vi "Menu_ItemName.vi"(7 "Ctrl":string, 8 "error in (no error)":errorcluster, 10 "DB Ref":T1, 11 "String":string) -> (0 "error out":errorcluster)   [LabVIEW 2017, in "tagdb-UIStateExpr Operations.lvlib"]
uses:
  tagdb-UIStateExpr Operations.lvlib
  <userlib>/_NEVSTOP/TagDB/Typedef/TagDB.ctl
  00d0da00-135c-4b50-b029-f1f1f0d03544.vi
  4c542a80-f847-4821-836c-1c9f0a826a9d.vi
  00d0da00-135c-4b50-b029-f1f1f0d03544.vi/1b47866c-8e2d-43a7-815f-8cf18635e5a1.vi
  4c542a80-f847-4821-836c-1c9f0a826a9d.vi/1b47866c-8e2d-43a7-815f-8cf18635e5a1.vi
  <userlib>/_NEVSTOP/TagDB/_Support/Change Detector/TagDB dbChanged.vi
  <userlib>/_NEVSTOP/TagDB/_Support/Error/_Clear Errors.vi
  00d0da00-135c-4b50-b029-f1f1f0d03544.vi/1b47866c-8e2d-43a7-815f-8cf18635e5a1.vi/29b2ea6d-6d7f-4e4a-ad31-a5cb760462c7.vi
  <userlib>/_NEVSTOP/TagDB/API/TagDB-Status.vi
  4c542a80-f847-4821-836c-1c9f0a826a9d.vi/1b47866c-8e2d-43a7-815f-8cf18635e5a1.vi/29b2ea6d-6d7f-4e4a-ad31-a5cb760462c7.vi
  <userlib>/_NEVSTOP/TagDB/_Support/Change Detector/TagDB ChangeFlag.vi
  <userlib>/_NEVSTOP/TagDB/_Support/DataAccess/_NameCacher.vi
  <userlib>/_NEVSTOP/TagDB/_Support/Error/_[error50002]Invalid DataType.vi
  <userlib>/_NEVSTOP/TagDB/_Support/Error/_[error50000]Invalid DB REF.vi
  <userlib>/_NEVSTOP/TagDB/_Support/DataAccess/TagDB Ref to DVR.vi
  <userlib>/_NEVSTOP/TagDB/_Support/URL/TRIM-BOTH-SPACE.vi
  <userlib>/_NEVSTOP/TagDB/_Support/Error/_Build Error Cluster.vi
  <userlib>/_NEVSTOP/TagDB/TagDB.lvlib
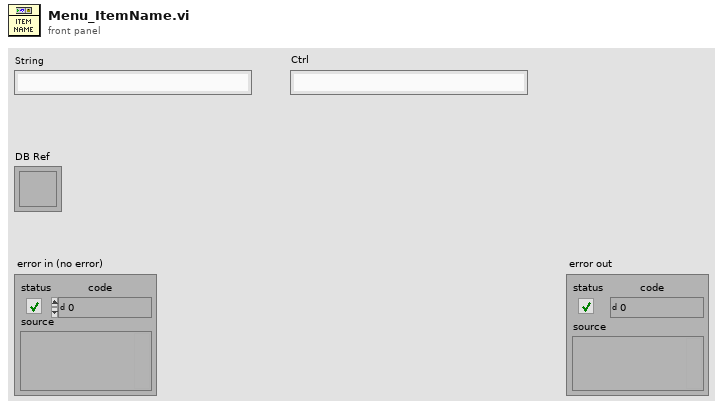
[diagram p1: front panel]
types:
  T1 = typedef "TagDB.lvlib/TagDB.ctl" = refnum<k1>
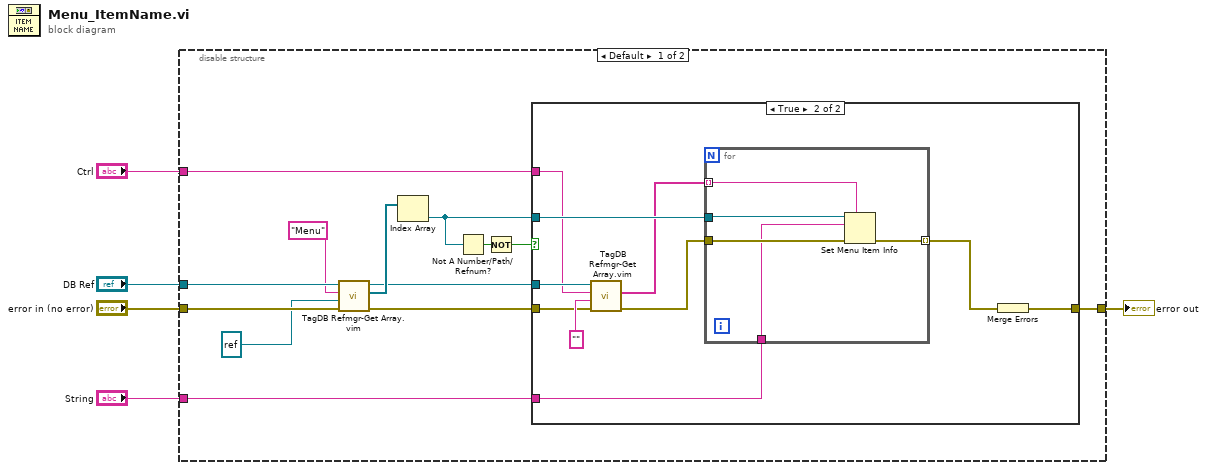
[diagram p0: block diagram]
diagram:
  n1 = disable-structure shown="Default" {
    disable-tunnel: "error in (no error)" -> [w18 w35]
    disable-tunnel: "DB Ref" -> [w17 _]
    disable-tunnel: "Ctrl" -> [w12 _]
    disable-tunnel: [w11 w35] -> w2
    disable-tunnel: "String" -> [w9 _]
    frame condition #0 (active) {
      n2 = call "TagDB Refmgr-Get Array.vim"("error in (no error)"=w18, "Type"=refnum<k9> refnum ("menu reference"), "RegExp"="Menu", "DB Ref"=w17) -> ("error out"=w10:errorcluster, "References"=w14:refnum<k9>[], "DB Ref(dup)"=w13:T1)  [unwired: 4 in, 1 out]
      n3 = Index Array(array=w14) -> (element=w6:refnum<k9>)  [unwired: 1 in]
      n4 = Not A Number/Path/Refnum?(number/path/refnum=w6) -> (NaN/Path/Refnum?=w8:bool)
      n5 = Not(x=w8) -> (.not. x?=w7:bool)
      n6 = case shown="True" w7 {
        tunnel: w13 -> [_ w29]
        tunnel: w6 -> [_ w28]
        tunnel: w12 -> [_ w26]
        tunnel: [w19 w23] -> w11
        tunnel: w10 -> [w19 w22]
        tunnel: w9 -> [_ w20]
        frame False {
        }
        frame True {
          n7 = call "TagDB Refmgr-Get Array.vim"("error in (no error)"=w22, "Type"="" ("RegExp"), "RegExp"=w26, "DB Ref"=w29) -> ("error out"=w21:errorcluster, "References"=w25:string[])  [unwired: 4 in, 2 out]
          n8 = for {
            tunnel: w28 -> [w34]
            tunnel: w25 -> [w33] mode=indexing
            tunnel: w21 -> [w32]
            tunnel: [w31] -> w24 mode=indexing
            tunnel: w20 -> [w30]
            n9 = Set Menu Item Info(7:w33, 8:w32, 10:w30, 11:w34) -> (0:w31:errorcluster)  [unwired: 3 in, 1 out]
          }
          n10 = Merge Errors(w24) -> (w23:errorcluster)
        }
      }
    }
    frame condition #1 {
    }
  }
  "error out" <- w2
